vi "FRCts20_Backend_API_Comment.vi"(8 "error in (no error)":errorcluster, 10 "Command":T1="GetNote", 11 "Note In":T2) -> (0 "error out":errorcluster, 2 "Status":string, 3 "Note Out":T2)   [LabVIEW 2014, in "FRCts20_Backend_Engine.lvlib" / "FRCts20_Backend_API.lvlib"]
doc: "This API call returns all information about a selected note, as part of a request. At present, it does not enforce the request index field (that is, the requested note must be part of the requested request)."
uses:
  FRCts20_Backend_API.lvlib
  Notes.ctl
  ApiReturn.ctl
  NotesRoot.ctl
  FRCts20_Backend_API_Command_Note.ctl
  FRCts20_Backend_FGVOperation.ctl
  FRCts20_Backend_Engine.lvlib
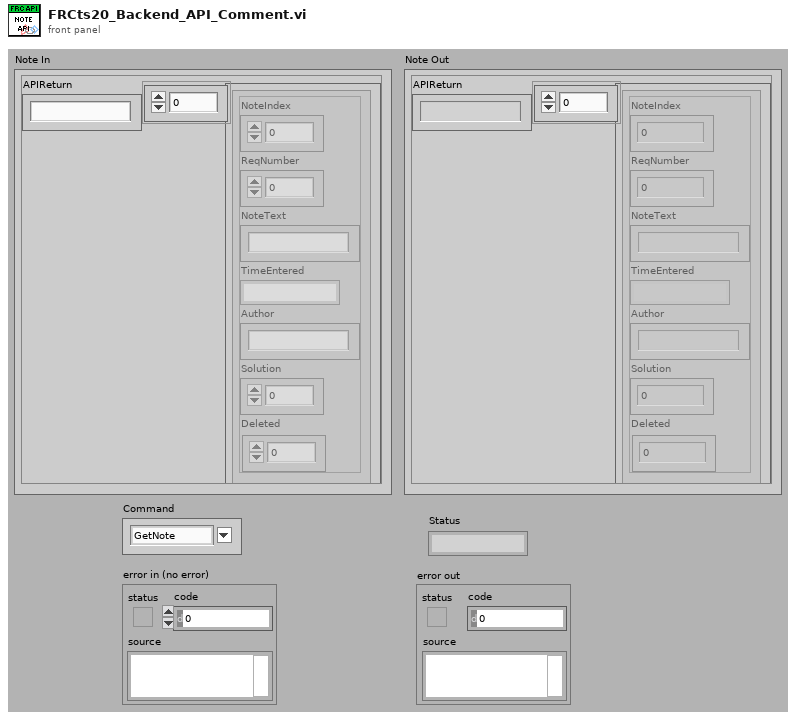
[diagram p1: front panel]
types:
  T1 = typedef "FRCts20_Backend_Engine.lvlib/FRCts20_Backend_API.lvlib/FRCts20_Backend_API_Command_Note.ctl" = string
  T2 = typedef "FRCts20_Backend_Engine.lvlib/FRCts20_Backend_API.lvlib/Notes.ctl" = cluster{"APIReturn":T3, "NotesRoot":T4}
  T3 = typedef "FRCts20_Backend_Engine.lvlib/FRCts20_Backend_API.lvlib/ApiReturn.ctl" = string
  T4 = typedef "FRCts20_Backend_Engine.lvlib/FRCts20_Backend_API.lvlib/NotesRoot.ctl" = cluster{"NoteIndex":u32, "ReqNumber":i32, "NoteText":string, "TimeEntered":string, "Author":string, "Solution":i32, "Deleted":i32}[]
  T5 = typedef "FRCts20_Backend_Engine.lvlib/FRCts20_Backend_FGVOperation.ctl" = enum16{"Initialize", "EnqueueMessage", "EnqueueDataReturn", "FlushMessage", "FlushDataReturn"}
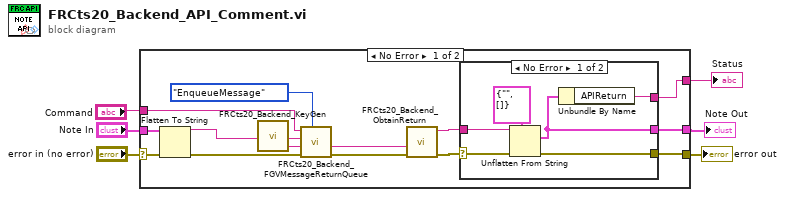
[diagram p0: block diagram]
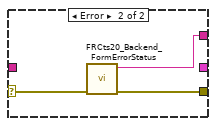
[diagram p2: hidden frame]
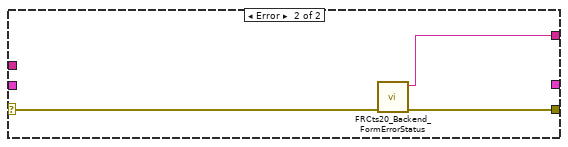
[diagram p3: hidden frame]
diagram:
  n1 = case shown="No Error" "error in (no error)" {
    selector: "error in (no error)" -> [w19 w32]
    tunnel: [w13 w31] -> w5
    tunnel: [w7 w30] -> w4
    tunnel: [w11 _] -> w3
    tunnel: "Command" -> [w10 _]
    tunnel: "Note In" -> [w9 _]
    frame No Error {
      n2 = Flatten To String(anything=w9, error in (no error)=w19) -> (data string=w20:string, error out=w18:errorcluster)  [unwired: 2 in, 1 out]
      n3 = call "FRCts20_Backend_KeyGen.vi"() -> ("Keygen"=w17:string)  [unwired: 27 in]
      n4 = call "FRCts20_Backend_FGVMessageReturnQueue.vi"("Operation"=FRCts20_Backend_FGVOperation."EnqueueMessage", "error in (no error)"=w18, "Key"=w17, "Message Value"=w20, "Message Name"=w10) -> ("error out"=w15:errorcluster, "Key (Duplicate)"=w14:string)  [unwired: 5 in]
      n5 = call "FRCts20_Backend_ObtainReturn.vi"("error in (no error)"=w15, "Key"=w14) -> ("error out"=w8:errorcluster, "Message Value"=w12:string)  [unwired: 8 in]
      n6 = case shown="No Error" w8 {
        selector: w8 -> [w23 w29]
        tunnel: [w26 w27] -> w13
        tunnel: w12 -> [w25 _]
        tunnel: [w22 _] -> w11
        tunnel: [w21 w28] -> w7
        frame No Error {
          n7 = Unflatten From String(type=T2 {"APIReturn"="", "NotesRoot"=[]} ("Note Out 2"), binary string=w25, error in (no error)=w23) -> (value=w22:T2, error out=w26:errorcluster)  [unwired: 2 in, 1 out]
          n8 = Unbundle By Name(w22) -> ("APIReturn"=w21:T3)
        }
        frame Error {
          n9 = call "FRCts20_Backend_FormErrorStatus.vi"("error in (no error)"=w29) -> ("error out"=w27:errorcluster, "String"=w28:string)  [unwired: 9 in]
        }
      }
    }
    frame Error {
      n10 = call "FRCts20_Backend_FormErrorStatus.vi"("error in (no error)"=w32) -> ("error out"=w31:errorcluster, "String"=w30:string)  [unwired: 9 in]
    }
  }
  "error out" <- w5
  "Status" <- w4
  "Note Out" <- w3
